vi "Example_Clustering.vi"() -> ()   [LabVIEW 2009]
uses:
  <vilib>/addons/Machine Learning/Utilities/Riffle (matrix with labels).vi
  <vilib>/addons/Machine Learning/Utilities/ml_Neighborhood Graph_Para.ctl
  <vilib>/addons/Machine Learning/NILabs_MLT.lvlib
panel:
  in  "# of samples":i32=1000
  in  "Data set":enum16{"4 Gaussians", "4 Concentric circles"}(ring)
  in  "# of clusters (k)":i32=4
  out "Rand index":dbl=0.9610930930930931
  out "Data":cluster{"X":dbl[], "Y":dbl[]}[](graph)
  out "Learned structure of the data":cluster{"X":dbl[], "Y":dbl[]}[](graph)=[{"X"=[-1.0121327456038078, -0.9492629822812026, 1.0125890329974099, 1.056230690770254], "Y"=[-1.092002490225518, 0.9282420227490457, -0.9853641035450806, 1.0320014347314106]}, {"X"=[], "Y"=[]}, {"X"=array[244 elements], "Y"=array[244 elements]}, {"X"=array[262 elements], "Y"=array[262 elements]}, {"X"=array[250 elements], "Y"=array[250 elements]}, {"X"=array[244 elements], "Y"=array[244 elements]}, {"X"=[], "Y"=[]}, {"X"=[], "Y"=[]}, {"X"=[], "Y"=[]}, {"X"=[], "Y"=[]}]
  in  "Algorithm":T1(ring)=enum."k-Means"
  out "Time (ms)":u32=6
  # "Introduction:\nA list of clustering algorithms can be selected to learn the structure of three data sets. The three data sets have different cluster structures, thereby for each of them some algorithms are sucessful in discovery of clusters while the others are not."
  # "(Samples are overlain with ground truth class labels.)"
  # "(Samples are overlain with class labels assgned by the algorithm.)"
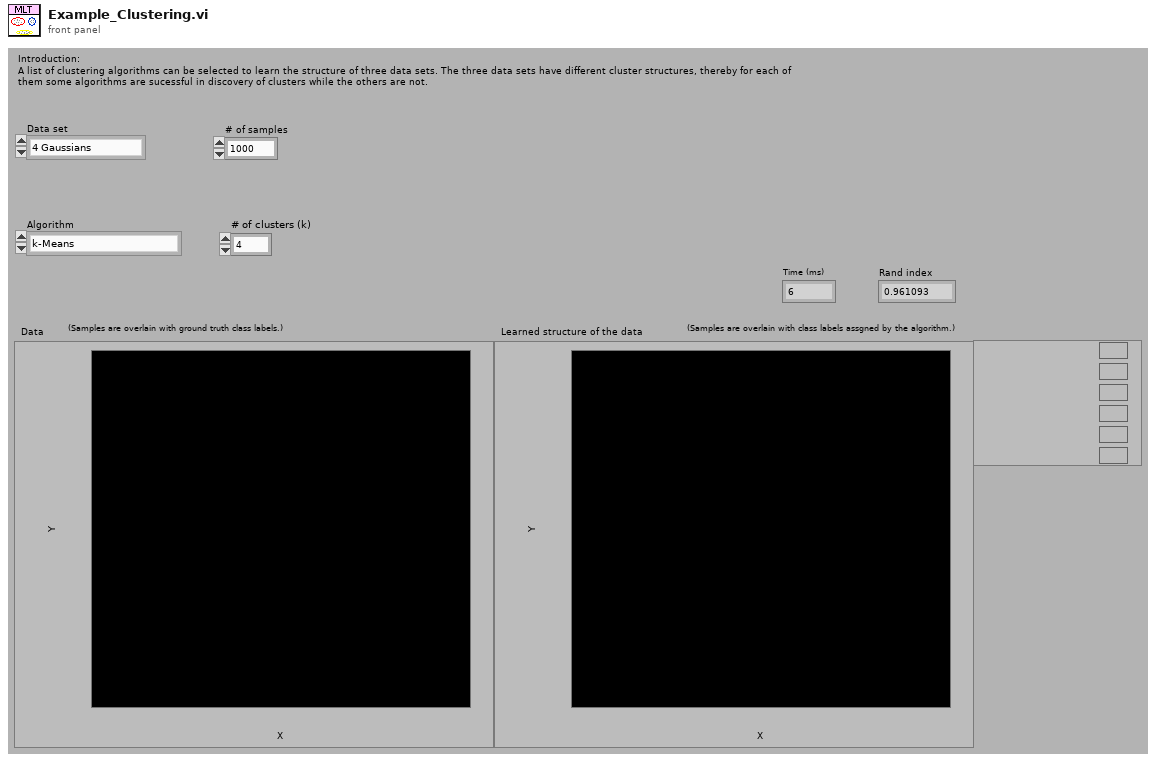
[diagram p1: front panel]
types:
  T1 = enum16{"Fuzzy C-Means Clustering", "Gaussian Mixture Models", "Hierarchical Clustering", "k-Means", "k-Medians", "k-Medoids", "Spectral Clustering", "Vector Quantization"}
  T2 = enum16{"Single Linkage", "Complete Linkage", "Average Linkage"}
  T3 = enum16{"Unnormalized Spectral Clustering", "Normalized Spectral Clustering"}
  T4 = typedef "NILabs_MLT.lvlib/ml_Neighborhood Graph_Para.ctl" = cluster{"algorithm":enum16{"eps-Neighborhood Graph", "k-Nearest Neighbor Graph", "Mutual k-Nearest Neighbor Graph"}, "k":i32, "eps":dbl}
  T5 = cluster{"Distance VI":refnum<vi>, "delta":dbl, "Neighborhood Graph Para ":T4}
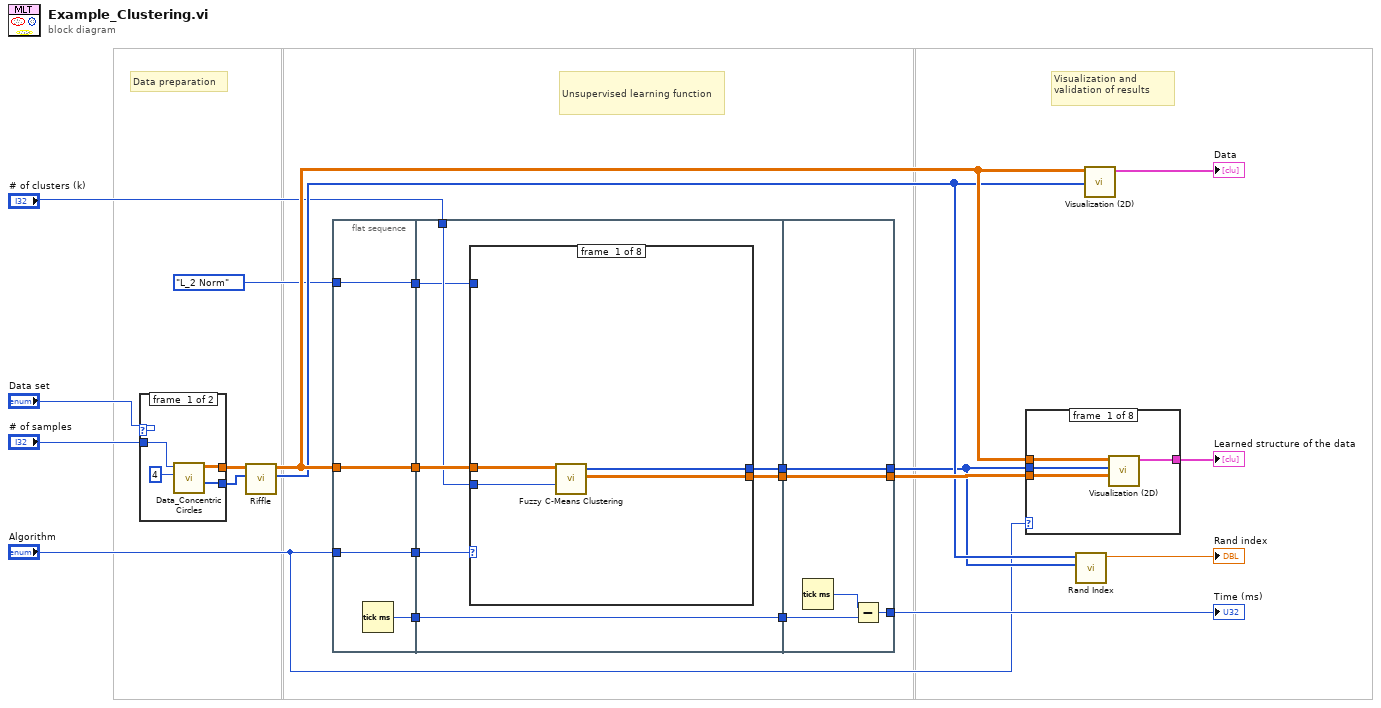
[diagram p0: block diagram]
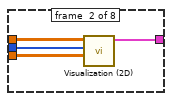
[diagram p2: hidden frame]
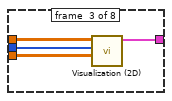
[diagram p3: hidden frame]
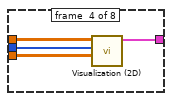
[diagram p4: hidden frame]
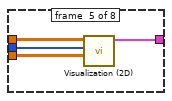
[diagram p5: hidden frame]
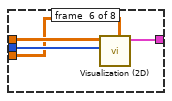
[diagram p6: hidden frame]
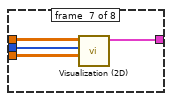
[diagram p7: hidden frame]
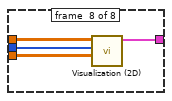
[diagram p8: hidden frame]
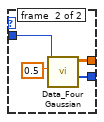
[diagram p9: hidden frame]
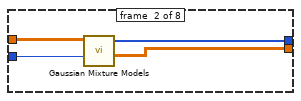
[diagram p10: hidden frame]
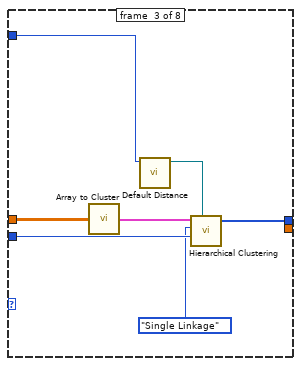
[diagram p11: hidden frame]
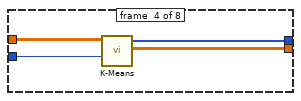
[diagram p12: hidden frame]
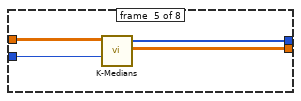
[diagram p13: hidden frame]
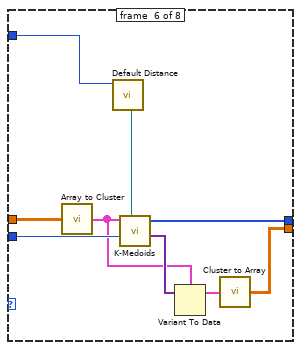
[diagram p14: hidden frame]
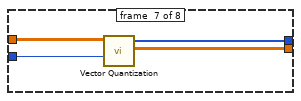
[diagram p15: hidden frame]
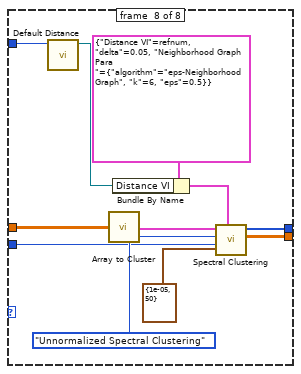
[diagram p16: hidden frame]
diagram:
  # "Visualization and validation of results"
  # "Unsupervised learning function"
  # "Data preparation"
  n1 = case shown="\"4 Concentric circles\"" "Data set" {
    tunnel: [w24 w30] -> w16
    tunnel: [w23 w29] -> w15
    tunnel: "# of samples" -> [w26 w28]
    frame #0 {
      n2 = call "Data_Concentric Circles.vi"("# of circles"=4, "# of points"=w26) -> ("Classes"=w23:i32[], "Data"=w24:dbl[][])  [unwired: 8 in]
    }
    frame #1 {
      n3 = call "Data_Four Gaussian.vi"("noise amplitude"=0.5, "# of points"=w28) -> ("Classes"=w29:i32[], "Data"=w30:dbl[][])  [unwired: 8 in]
    }
  }
  n4 = call-poly <vilib>:"Riffle.vi"("Labels"=w15, "Data"=w16) -> ("Riffled{Labels}"=w9:i32[], "Riffled{Data}"=w11:dbl[][])  [unwired: 6 in, 2 out]
  n5 = flat-sequence {
    tunnel: [w34] -> w22
    tunnel: [w33] -> w21
    tunnel: w11 -> [w33]
    tunnel: enum16{"L_1 Norm", "L_2 Norm", "L_inf Norm"}."L_2 Norm" ("Distance norm type") -> [w32]
    tunnel: [w32] -> w4
    tunnel: [w31] -> w3
    tunnel: "Algorithm" -> [w31]
    tunnel: [w41] -> w20
    tunnel: [w40] -> w19
    tunnel: w22 -> [w40]
    tunnel: w21 -> [w39]
    tunnel: [w38] -> w13
    tunnel: "# of clusters (k)" -> [w37]
    tunnel: w4 -> [w36]
    tunnel: w3 -> [w35]
    tunnel: [w93] -> w17
    tunnel: w20 -> [w93]
    tunnel: w19 -> [w92]
    tunnel: [w90] -> w18
    tunnel: [w89] -> w8
    tunnel: w13 -> [w89]
    frame #0 {
      n6 = Tick Count (ms)() -> (millisecond timer value=w34:u32)
    }
    frame #1 {
      n7 = case shown="\"Hierarchical Clustering\"" w35 {
        tunnel: [w44 w47 _ w58 w62 w69 w74 w80] -> w41
        tunnel: w39 -> [w45 w49 w55 w60 w64 w70 w77 w79]
        tunnel: [w43 w48 w56 w59 w61 w72 w75 w81] -> w38
        tunnel: w37 -> [w42 w46 w54 w57 w63 w71 w76 w78]
        tunnel: w36 -> [_ _ w50 _ _ w65 _ w82]
        frame #0 {
          n8 = call <vilib>:"Fuzzy C-Means Clustering.vi"("# of classes"=w42, "Data samples"=w45) -> ("Centroids"=w44:dbl[][], "Class labels"=w43:i32[])  [unwired: 6 in, 2 out]
        }
        frame #1 {
          n9 = call <vilib>:"Gaussian Mixture Models.vi"("# of classes"=w46, "Data samples"=w49) -> ("Centroids"=w47:dbl[][], "Class labels"=w48:i32[])  [unwired: 5 in, 3 out]
        }
        frame #2 {
          n10 = call <vilib>:"Array to Cluster.vi"("Data in Array"=w55) -> ("Data in Cluster"=w53:cluster{"Sample":dbl[]}[])
          n11 = call <vilib>:"Default Distance.vi"("distance norm type"=w50) -> ("Distance VI"=w51:refnum<vi>)  [unwired: 9 in, 1 out]
          n12 = call <vilib>:"Hierarchical Clustering.vi"("Distance VI"=w51, "# of classes"=w54, "Linkage type"=T2."Single Linkage", "Data samples"=w53) -> ("Class labels"=w56:i32[])  [unwired: 5 in, 2 out]
        }
        frame #3 {
          n13 = call <vilib>:"K-Means.vi"("# of classes"=w57, "Data samples"=w60) -> ("Centroids"=w58:dbl[][], "Class labels"=w59:i32[])  [unwired: 7 in, 1 out]
        }
        frame #4 {
          n14 = call <vilib>:"K-Medians.vi"("# of classes"=w63, "Data samples"=w64) -> ("Centroids"=w62:dbl[][], "Class labels"=w61:i32[])  [unwired: 7 in, 1 out]
        }
        frame #5 {
          n15 = call <vilib>:"Array to Cluster.vi"("Data in Array"=w70) -> ("Data in Cluster"=w67:cluster{"Sample":dbl[]}[])
          n16 = call <vilib>:"Default Distance.vi"("distance norm type"=w65) -> ("Distance VI"=w73:refnum<vi>)  [unwired: 9 in, 1 out]
          n17 = call <vilib>:"K-Medoids.vi"("Distance VI"=w73, "# of classes"=w71, "Data samples"=w67) -> ("Centroids"=w68:variant[], "Class labels"=w72:i32[])  [unwired: 5 in, 2 out]
          n18 = Variant To Data(Variant=w68, type=w67) -> (data=w66:cluster{"Sample":dbl[]}[])  [unwired: 1 in, 1 out]
          n19 = call <vilib>:"Cluster to Array.vi"("Data in Cluster"=w66) -> ("Data in Array"=w69:dbl[][])
        }
        frame #6 {
          n20 = call <vilib>:"Vector Quantization.vi"("# of classes"=w76, "Data samples"=w77) -> ("Centroids"=w74:dbl[][], "Class labels"=w75:i32[])  [unwired: 7 in, 1 out]
        }
        frame #7 {
          n21 = call <vilib>:"Default Distance.vi"("distance norm type"=w82) -> ("Distance VI"=w85:refnum<vi>)  [unwired: 9 in, 1 out]
          n22 = call <vilib>:"Array to Cluster.vi"("Data in Array"=w79) -> ("Data in Cluster"=w87:cluster{"Sample":dbl[]}[])
          n23 = Bundle By Name(cluster=T5 {"Distance VI"=refnum, "delta"=0.05, "Neighborhood Graph Para "={"algorithm"=enum."eps-Neighborhood Graph", "k"=6, "eps"=0.5}} ("similarity parameters"), "Distance VI"=w85) -> (w86:T5)
          n24 = call <vilib>:"Spectral Clustering.vi"("stopping criteria"=cluster{"tolarence":dbl, "max iterations":i32} {"tolarence"=1e-05, "max iterations"=50}, "similarity parameters"=w86, "# of classes"=w78, "algorithm"=T3."Unnormalized Spectral Clustering", "Data samples"=w87) -> ("Similarity Matrix"=w80:dbl[][], "Class labels"=w81:i32[])  [unwired: 4 in, 1 out]
        }
      }
    }
    frame #2 {
      n25 = Tick Count (ms)() -> (millisecond timer value=w91:u32)
      n26 = Subtract(x=w91, y=w92) -> (x-y=w90:u32)
    }
  }
  n27 = case shown="\"Fuzzy C-Means Clustering\"" "Algorithm" {
    tunnel: w17 -> [w97 w101 w105 w109 w113 w114 w121 w125]
    tunnel: [w96 w100 w104 w108 w112 w117 w120 w124] -> w14
    tunnel: w11 -> [w95 w99 w103 w107 w111 w116 w119 w123]
    tunnel: w8 -> [w94 w98 w102 w106 w110 w115 w118 w122]
    frame #0 {
      n28 = call <vilib>:"Visualization (2D).vi"("Centroids"=w97, "Class labels"=w94, "Data samples"=w95) -> ("XY Graph"=w96:cluster{"X":dbl[], "Y":dbl[]}[])  [unwired: 7 in, 1 out]
    }
    frame #1 {
      n29 = call <vilib>:"Visualization (2D).vi"("Centroids"=w101, "Class labels"=w98, "Data samples"=w99) -> ("XY Graph"=w100:cluster{"X":dbl[], "Y":dbl[]}[])  [unwired: 7 in, 1 out]
    }
    frame #2 {
      n30 = call <vilib>:"Visualization (2D).vi"("Centroids"=w105, "Class labels"=w102, "Data samples"=w103) -> ("XY Graph"=w104:cluster{"X":dbl[], "Y":dbl[]}[])  [unwired: 7 in, 1 out]
    }
    frame #3 {
      n31 = call <vilib>:"Visualization (2D).vi"("Centroids"=w109, "Class labels"=w106, "Data samples"=w107) -> ("XY Graph"=w108:cluster{"X":dbl[], "Y":dbl[]}[])  [unwired: 7 in, 1 out]
    }
    frame #4 {
      n32 = call <vilib>:"Visualization (2D).vi"("Centroids"=w113, "Class labels"=w110, "Data samples"=w111) -> ("XY Graph"=w112:cluster{"X":dbl[], "Y":dbl[]}[])  [unwired: 7 in, 1 out]
    }
    frame #5 {
      n33 = call <vilib>:"Visualization (2D).vi"("Neighborhood Graph"=w114, "Class labels"=w115, "Data samples"=w116) -> ("XY Graph"=w117:cluster{"X":dbl[], "Y":dbl[]}[])  [unwired: 7 in, 1 out]
    }
    frame #6 {
      n34 = call <vilib>:"Visualization (2D).vi"("Centroids"=w121, "Class labels"=w118, "Data samples"=w119) -> ("XY Graph"=w120:cluster{"X":dbl[], "Y":dbl[]}[])  [unwired: 7 in, 1 out]
    }
    frame #7 {
      n35 = call <vilib>:"Visualization (2D).vi"("Centroids"=w125, "Class labels"=w122, "Data samples"=w123) -> ("XY Graph"=w124:cluster{"X":dbl[], "Y":dbl[]}[])  [unwired: 7 in, 1 out]
    }
  }
  "Learned structure of the data" <- w14
  n36 = call <vilib>:"Rand Index.vi"("Class labels 2"=w8, "Class labels 1"=w9) -> ("Rand Index"=→"Rand index":dbl)  [unwired: 8 in, 1 out]
  n37 = call <vilib>:"Visualization (2D).vi"("Class labels"=w9, "Data samples"=w11) -> ("XY Graph"=→"Data":cluster{"X":dbl[], "Y":dbl[]}[])  [unwired: 8 in, 1 out]
  "Time (ms)" <- w18
